vi "Init.vi"(3 "Container State":T4 caption="容器状态", 4 "Previous State":variant caption="前期状态", 5 "Previous Version":T3 caption="前期版本") -> (2 "Current State":T1 caption="当前状态")   [LabVIEW 2011, in "WaveFormGraph.xctl"]
uses:
  WaveFormGraph.xctl
  State.ctl
  F:/Program Files/National Instruments/LabVIEW 2011/resource/importtools/Common/Event/NISAST Event.lvclass
  CursorPosQueueCluster.ctl
  <vilib>/_xctls/Container State.ctl
  <vilib>/_xctls/Version.ctl
  <vilib>/_xctls/XControlSupport.lvlib
panel:
  in  "Default Indicator State":T1 caption="默认显示控件状态"
  in  "Default Control State":T1 caption="默认输入控件状态"
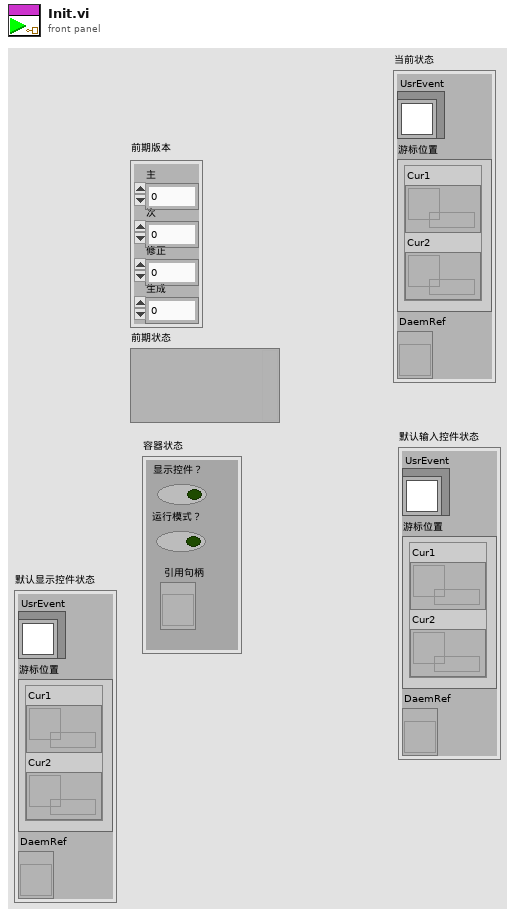
[diagram p1: front panel]
types:
  T1 = typedef "WaveFormGraph.xctl/State.ctl" = cluster{"UsrEvent":refnum<class "NISAST Event.lvclass">, "游标位置":T2, "DaemRef":refnum<vi>}
  T2 = typedef "CursorPosQueueCluster.ctl" = cluster{"Cur1":refnum<queue>, "Cur2":refnum<queue>}
  T3 = typedef "XControlSupport.lvlib/Version.ctl" = cluster{"Major":u16, "Minor":u16, "Fix":u16, "Build":u16}
  T4 = typedef "XControlSupport.lvlib/Container State.ctl" = cluster{"Indicator?":bool, "Run Mode?":bool, " Refnum":refnum<vi>}
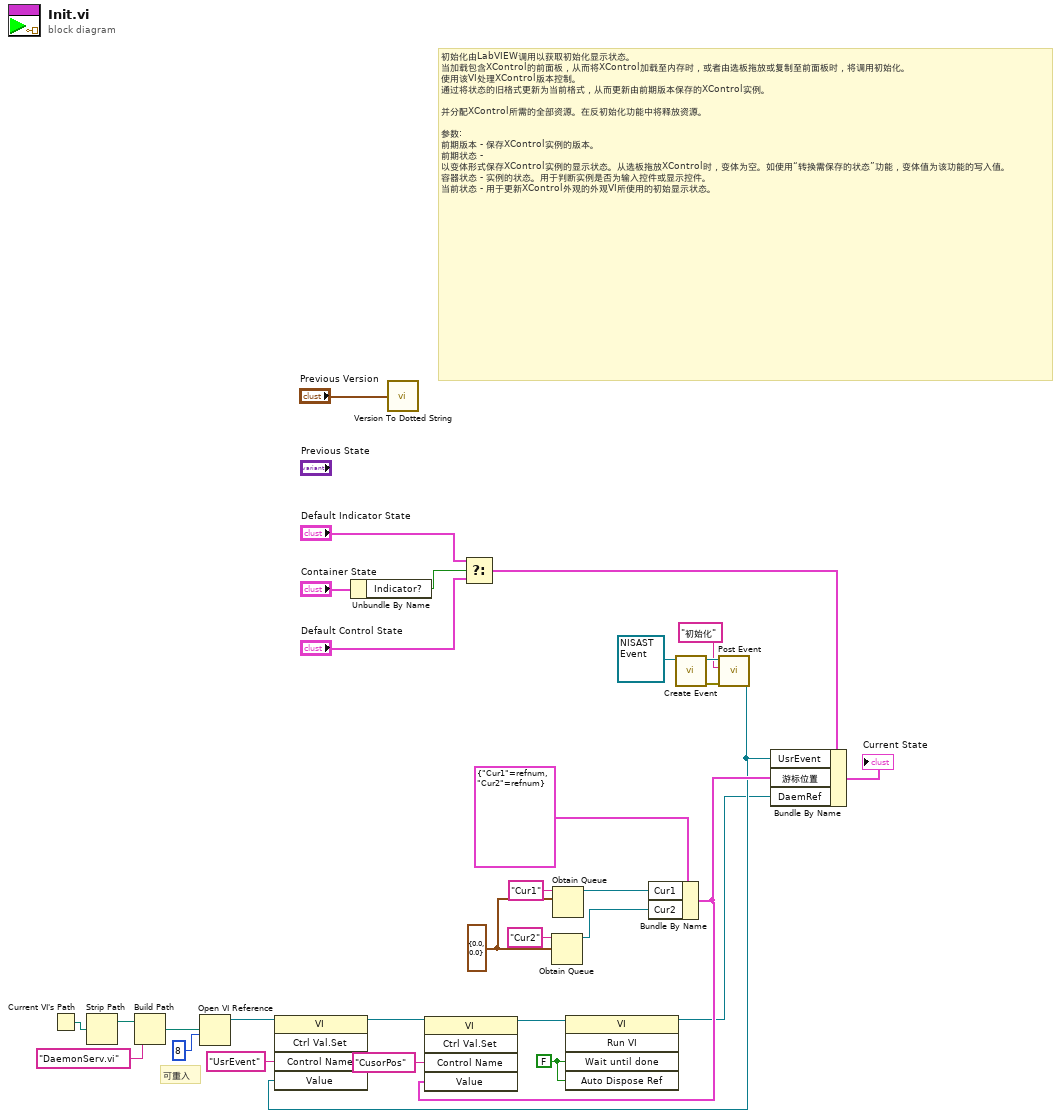
[diagram p0: block diagram]
diagram:
  w1 = FALSE ("结束前等待")
  w19 = cluster{"X":dbl, "Y":dbl} {"X"=0.0, "Y"=0.0} ("Position")
  # "可重入"
  # "初始化由LabVIEW调用以获取初始化显示状态。\n当加载包含XControl的前面板，从而将XControl加载至内存时，或者由选板拖放或复制至前面板时，将调用初始化。\n使用该VI处理XControl版本控制。\n通过将状态的旧格式更新为当前格式，从而更新由前期版本保存的XControl实例。\n\n并分配XControl所需的全部资源。在反初始化功能中将释放资源。\n\n参数: \n前期版本 - 保存XControl实例的版本。\n前期状态 - 以变体形式保存XControl实例的显示状态。从选板拖放XControl时，变体为空。如使用“转换需保存的状态”功能，变体值为该功能的写入值。\n容器状态 - 实例的状态。用于判断实例是否为输入控件或显示控件。\n当前状态 - 用于更新XControl外观的外观VI所使用的初始显示状态。"
  n1 = Current VI's Path() -> (path=w13:path)
  n2 = Strip Path(path=w13) -> (stripped path=w14:path)  [unwired: 1 out]
  n3 = Build Path(base path=w14, name or relative path="DaemonServ.vi" ("名称或相对路径")) -> (appended path=w11:path)
  n4 = Open VI Reference(vi path=w11, options=8 ("选项")) -> (vi reference=w9:refnum<vi>)  [unwired: 4 in, 1 out]
  n5 = Unbundle By Name("Container State") -> ("Indicator?"=w28:bool)
  n6 = call <vilib>:"Version To Dotted String.vi"("Version"="Previous Version") -> ()  [unwired: 1 out]
  n7 = Select(t="Default Indicator State", s=w28, f="Default Control State") -> (s? t:f=w26:T1)
  n8 = Obtain Queue(name (unnamed)="Cur2" ("名称（未命名）"), element data type=w19) -> (queue out=w15:refnum<queue>)  [unwired: 3 in, 2 out]
  n9 = Obtain Queue(name (unnamed)="Cur1" ("名称（未命名）"), element data type=w19) -> (queue out=w16:refnum<queue>)  [unwired: 3 in, 2 out]
  n10 = Bundle By Name(cluster=T2 {"Cur1"=refnum, "Cur2"=refnum} ("游标位置"), "Cur1"=w16, "Cur2"=w15) -> (w5:T2)
  n11 = call-dynamic "Create Event.vi"("Event in"=refnum<class "NISAST Event.lvclass"> refnum ("NISAST Event.lvclass")) -> ("error out"=w21:errorcluster, "Event out"=w23:refnum<class "NISAST Event.lvclass">)  [unwired: 8 in, 1 out]
  n12 = call-dynamic "Post Event.vi"("error in (no error)"=w21, "Event Name"="初始化", "Event in"=w23) -> ("Event out"=w4:refnum<class "NISAST Event.lvclass">)  [unwired: 7 in, 1 out]
  n13 = invoke class="VI" method="Ctrl Val.Set"(reference=w9, "Control Name"="UsrEvent" ("控件名"), "Value"=w4) -> (reference out=w8:refnum<vi>)  [unwired: 2 in, 4 out]
  n14 = invoke class="VI" method="Ctrl Val.Set"(reference=w8, "Control Name"="CusorPos" ("控件名"), "Value"=w5) -> (reference out=w3:refnum<vi>)  [unwired: 2 in, 4 out]
  n15 = invoke class="VI" method="Run VI"(reference=w3, "Wait until done"=w1, "Auto Dispose Ref"=w1) -> (reference out=w2:refnum<vi>)  [unwired: 2 in, 4 out]
  n16 = Bundle By Name(cluster=w26, "UsrEvent"=w4, "游标位置"=w5, "DaemRef"=w2) -> (→"Current State":T1)
